vi "Reader.vi"() -> (0 "error out":errorcluster)   [LabVIEW 2021]
uses:
  Zenoh.lvclass/Zenoh.ctl
  Wrappers/Poll Raw Wrapper.vi
  Core/Read Double.vi/4c4e9aed-29a9-49a4-ae79-bb096e87db4b.vi
  Core/Read Double.vi/4c4e9aed-29a9-49a4-ae79-bb096e87db4b.vi/c28b0ead-42ad-4072-80a2-aca7f2bd7ce3.vi
  Core/Read Double.vi/4c4e9aed-29a9-49a4-ae79-bb096e87db4b.vi/48104490-ec73-4168-8754-ff252ec03617.vi
  <vilib>/CIF Foundation/CIF Utilities/DataTypes/SubVIs/DataTypes Error.vi
  Core/Read Double.vi/4c4e9aed-29a9-49a4-ae79-bb096e87db4b.vi/543c0f61-77eb-4f29-b175-1688c1700ba4.vi
  <vilib>/CIF Foundation/CIF Utilities/Errors/Append Error Location.vi
  SubVIs/Get Zenoh Path.vi
  Zenoh.lvclass
panel:
  in  "Poll Rate (ms)":u32=100
  out "Read Value":dbl
  in  "stop":bool
  in  "key":string="myhome/kitchen/temp"
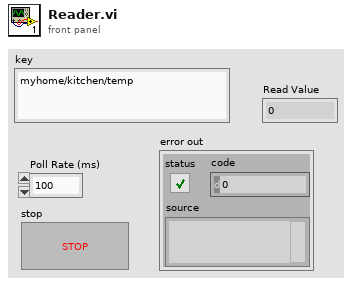
[diagram p1: front panel]
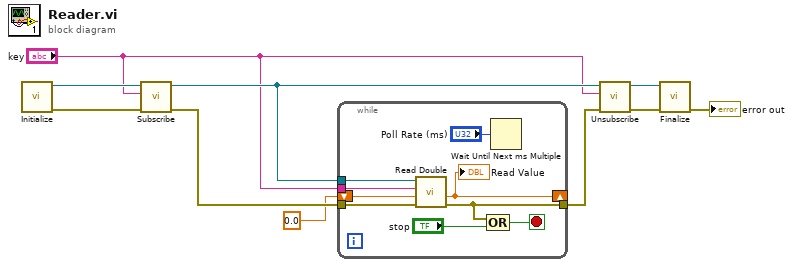
[diagram p0: block diagram]
diagram:
  n1 = call "Initialize.vi"() -> ("error out"=w10:errorcluster, "Zenoh out"=w9:refnum<class "Zenoh.lvclass">)  [unwired: 10 in]
  n2 = call "Subscribe.vi"("error in (no error)"=w10, "Key"="key", "Zenoh in"=w9) -> ("error out"=w3:errorcluster, "Zenoh out"=w8:refnum<class "Zenoh.lvclass">)  [unwired: 7 in]
  n3 = while {
    tunnel: w8 -> [w19]
    tunnel: "key" -> [w18]
    tunnel: w3 -> [w17]
    tunnel: [w13] -> w2
    shift-right: [w16] -> _
    shift-left: 0.0 ("Numeric Out") -> [w15]
    stop <- w11 stop-if-true
    n4 = call "Read Double.vi"("error in (no error)"=w17, "Numeric In"=w15, "Key"=w18, "Zenoh in"=w19) -> ("error out"=w13:errorcluster, "Numeric Out"=w16:dbl)  [unwired: 5 in, 1 out]
    "Read Value" <- w16
    n5 = Compound Arithmetic op=OR(w13, "stop") -> (w11:bool)
    n6 = Wait Until Next ms Multiple(millisecond multiple="Poll Rate (ms)") -> ()  [unwired: 1 out]
  }
  n7 = call "Unsubscribe.vi"("error in (no error)"=w2, "Key"="key", "Zenoh in"=w8) -> ("error out"=w6:errorcluster, "Zenoh out"=w5:refnum<class "Zenoh.lvclass">)  [unwired: 7 in]
  n8 = call "Finalize.vi"("error in (no error)"=w6, "Zenoh in"=w5) -> ("error out"=→"error out":errorcluster)  [unwired: 8 in, 1 out]
